vi "Nested Alias Unique.vi"(10 "Nested Alias":string, 11 "Self Actor":refnum<class "Self Actor.lvclass">) -> (0 "error out":errorcluster, 2 "Nested Alias Unique?":bool)   [LabVIEW 2021, in "jettl.lvlib" / "Self Actor.lvclass"]
uses:
  Self Actor.lvclass
  Self Actor.lvclass/Self Actor.ctl
  jettl.lvlib
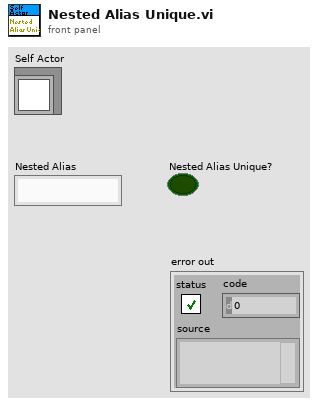
[diagram p1: front panel]
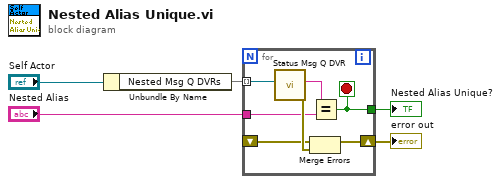
[diagram p0: block diagram]
diagram:
  n1 = Unbundle By Name("Self Actor") -> ("Nested Msg Q DVRs"=w1:set{refnum<data-value>})
  n2 = for {
    tunnel: w1 -> [w12] mode=indexing
    shift-right: [w10] -> w5
    shift-left: _ -> [w9]
    tunnel: "Nested Alias" -> [w7]
    tunnel: [w6] -> w3
    stop <- w6 stop-if-true
    n3 = call "Status Msg Q DVR.vi"("Msg Q DVR"=w12) -> ("error out"=w11:errorcluster, "Msg Q DVR Alias"=w8:string)  [unwired: 9 in]
    n4 = Merge Errors(w9, w11) -> (w10:errorcluster)
    n5 = Equal?(x=w8, y=w7) -> (x = y?=w6:bool)
  }
  "error out" <- w5
  "Nested Alias Unique?" <- w3
